vi "SwerveModuleReadData.vi"(10 "NT Name (Errors)":string, 11 "NT Name (Details)":string) -> (0 "Shifter State":string, 1 "Drive Velocity":dbl format="%.1f", 2 "Drive Temperature":dbl, 3 "Azimuth Position":dbl format="%.1f", 4 "Shifter Failure":T1, 5 "Drive Overheating":T1, 7 "Azimuth Fault":T1)   [LabVIEW 2020]
uses:
  <vilib>/Rock Robotics/Network Tables/NT Read Numeric Array.vi
  <vilib>/Rock Robotics/Network Tables/NT Read Boolean Array.vi
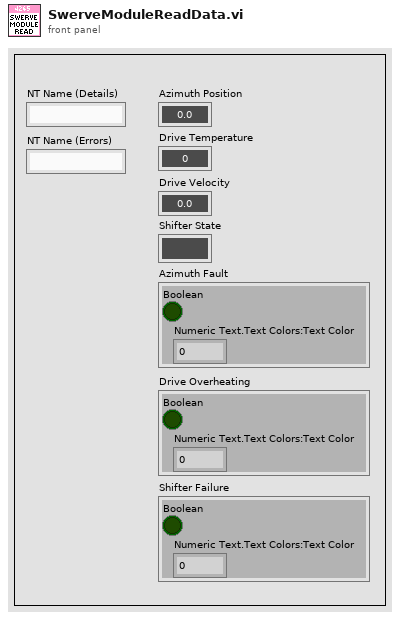
[diagram p1: front panel]
types:
  T1 = cluster{"Boolean":bool, "Numeric Text.Text Colors:Text Color":u32}
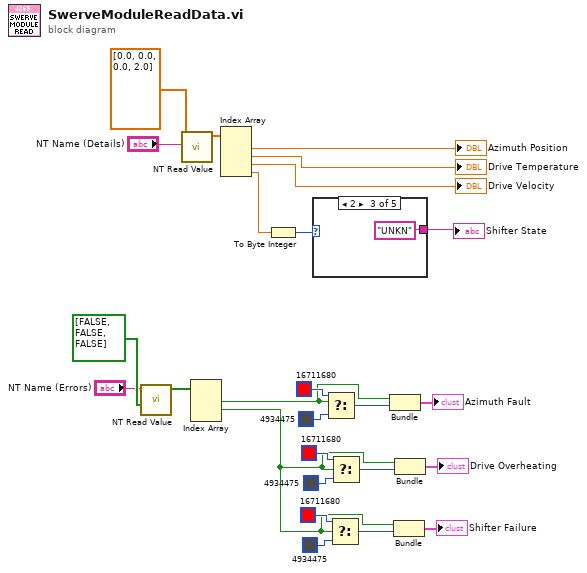
[diagram p0: block diagram]
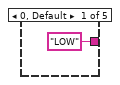
[diagram p2: hidden frame]
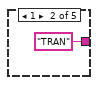
[diagram p3: hidden frame]
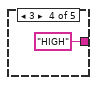
[diagram p4: hidden frame]
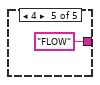
[diagram p5: hidden frame]
diagram:
  n1 = call-poly <vilib>:"NT Read Value.vi"("Default Value"=bool[] [FALSE, FALSE, FALSE], "Name"="NT Name (Errors)") -> ("Boolean Array"=w17:bool[])  [unwired: 8 in, 1 out]
  n2 = call-poly <vilib>:"NT Read Value.vi"("Default Value"=dbl[] [0.0, 0.0, 0.0, 2.0], "Name"="NT Name (Details)") -> ("Numeric Array"=w23:dbl[])  [unwired: 8 in, 1 out]
  n3 = Index Array(array=w17) -> (element #1=w12:bool, element #2=w2:bool)  [unwired: 3 in, 1 out]
  n4 = Index Array(array=w23) -> (element #1=→"Azimuth Position":dbl, element #2=→"Drive Temperature":dbl, element #3=→"Drive Velocity":dbl, element #4=w19:dbl)  [unwired: 4 in]
  n5 = To Byte Integer(number=w19) -> (8bit integer=w18:i8)
  n6 = case shown="2" w18 {
    tunnel: ["LOW" "TRAN" "UNKN" "HIGH" "FLOW"] -> w20
    frame 0, Default {
    }
    frame 1 {
    }
    frame 2 {
    }
    frame 3 {
    }
    frame 4 {
    }
  }
  "Shifter State" <- w20
  n7 = Select(t=u32 16711680 ("Numeric Text.Text Colors:Text Color"), s=w12, f=u32 4934475 ("Numeric Text.Text Colors:Text Color")) -> (s? t:f=w13:u32)
  n8 = Select(t=u32 16711680 ("Numeric Text.Text Colors:Text Color"), s=w2, f=u32 4934475 ("Numeric Text.Text Colors:Text Color")) -> (s? t:f=w4:u32)
  n9 = Select(t=u32 16711680 ("Numeric Text.Text Colors:Text Color"), s=w2, f=u32 4934475 ("Numeric Text.Text Colors:Text Color")) -> (s? t:f=w8:u32)
  n10 = Bundle("Boolean"=w12, "Numeric Text.Text Colors:Text Color"=w13) -> (→"Azimuth Fault":T1)  [unwired: 1 in]
  n11 = Bundle("Boolean"=w2, "Numeric Text.Text Colors:Text Color"=w4) -> (→"Shifter Failure":T1)  [unwired: 1 in]
  n12 = Bundle("Boolean"=w2, "Numeric Text.Text Colors:Text Color"=w8) -> (→"Drive Overheating":T1)  [unwired: 1 in]
